vi "AeroProbeAppendPandT.vi"() -> ()   [LabVIEW 2013]
panel:
  out "appended array":dbl[][](array[numeric])
  in  "initialized array 2":dbl[](array[numeric])=array[8192 elements]
  in  "initialized array":dbl[](array[numeric])=array[8192 elements]
  in  "x*y":dbl[][](array[numeric])=array8192x5[40960 elements]
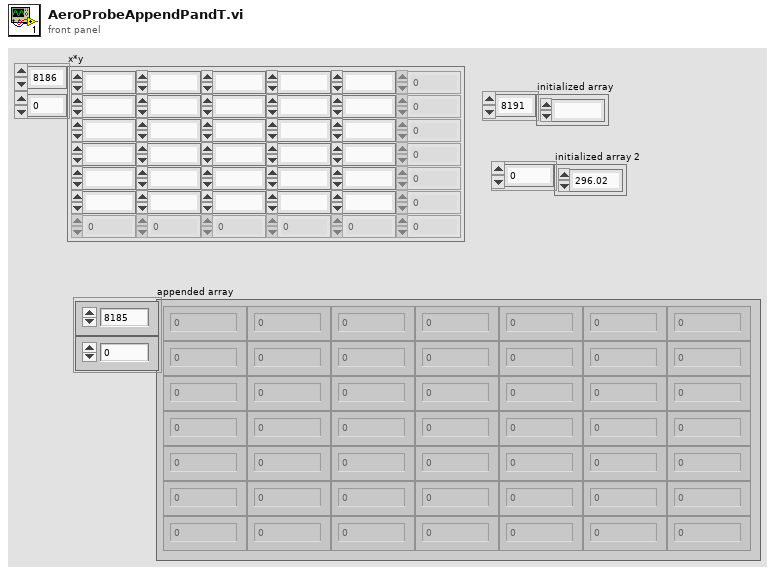
[diagram p1: front panel]
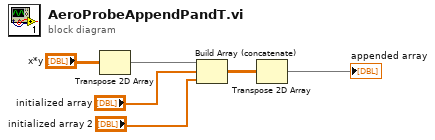
[diagram p0: block diagram]
diagram:
  n1 = Transpose 2D Array(2D array="x*y") -> (transposed array=w2:dbl[][])
  n2 = Build Array (concatenate)(w2, "initialized array", "initialized array 2") -> (w3:dbl[][])
  n3 = Transpose 2D Array(2D array=w3) -> (transposed array=→"appended array":dbl[][])
